vi "Close.vi"(8 "error in (no error)":errorcluster, 11 "Accelerometer Ref In":T1) -> (0 "error out":errorcluster)   [LabVIEW 2021, in "Accelerometer.lvlib"]
doc: "Closes the reference to accelerometer channels."
uses:
  <vilib>/myRIO/Instrument Drivers/Onboard Devices/Accelerometer/Accelerometer.lvlib
  <vilib>/myRIO/Instrument Drivers/Onboard Devices/Accelerometer/typedefs/Accelerometer Reference.ctl
  <vilib>/myRIO/Common/Instrument Driver Framework/Utilities/typedefs/myRIO Generic Hardware Reference.ctl
  <vilib>/myRIO/Common/Instrument Driver Framework/Utilities/typedefs/Hardware Version Enum.ctl
  <vilib>/myRIO/Common/Instrument Driver Framework/Utilities/typedefs/myRIO v1.0 Reference.ctl
  <vilib>/myRIO/Common/Instrument Driver Framework/Utilities/typedefs/Generic FPGA Reference.ctl
  <vilib>/myRIO/Common/Instrument Driver Framework/myRIO v1.0/Accelerometer/typedefs/Accelerometer Channels List.ctl
  <vilib>/myRIO/Common/Instrument Driver Framework/myRIO v1.0/Accelerometer/typedefs/Accelerometer Channels Enum.ctl
  <vilib>/myRIO/Common/Instrument Driver Framework/myRIO v1.0/Accelerometer/vis/myRIO v1.0 Unreserve Accelerometer.vi
  <vilib>/myRIO/Common/Instrument Driver Framework/roboRIO v1.0/Accelerometer/vis/roboRIO v1.0 Unreserve Accelerometer.vi
  <vilib>/myRIO/Common/Instrument Driver Framework/myRIO v1.0/Resource Manager/vis/myRIO v1.0 Unreserve Channel List.vi
  <vilib>/myRIO/Common/Instrument Driver Framework/myRIO v1.0/Accelerometer/vis/myRIO v1.0 Build MUX Configuration Accelerometer.vi
  <vilib>/myRIO/Common/Instrument Driver Framework/roboRIO v1.0/Resource Manager/vis/roboRIO v1.0 Unreserve Channel List.vi
  <vilib>/myRIO/Common/Instrument Driver Framework/roboRIO v1.0/Accelerometer/vis/roboRIO v1.0 Build MUX Configuration Accelerometer.vi
  <vilib>/myRIO/Common/Instrument Driver Framework/myRIO v1.0/Resource Manager/vis/myRIO v1.0 Unreserve Channel.vi
  <vilib>/myRIO/Common/Instrument Driver Framework/roboRIO v1.0/Resource Manager/vis/roboRIO v1.0 Unreserve Channel.vi
  <vilib>/myRIO/Common/Instrument Driver Framework/myRIO v1.0/Resource Manager/vis/myRIO v1.0 Build Mutex Name.vi
  <vilib>/myRIO/Common/Instrument Driver Framework/roboRIO v1.0/Resource Manager/vis/roboRIO v1.0 Build Mutex Name.vi
  <vilib>/myRIO/Common/Instrument Driver Framework/Utilities/vis/Configuration Manager.vi
  <vilib>/myRIO/Common/Instrument Driver Framework/Utilities/vis/IO Manager.vi
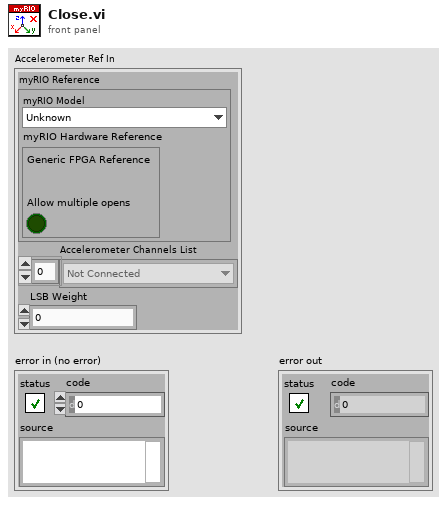
[diagram p1: front panel]
types:
  T1 = typedef "Accelerometer.lvlib/Accelerometer Reference.ctl" = cluster{"myRIO Reference":T2, "Accelerometer Channels List":T6, "LSB Weight":dbl}
  T2 = typedef "myRIO Generic Hardware Reference.ctl" = cluster{"myRIO Model":T3, "myRIO Hardware Reference":T4}
  T3 = typedef "Hardware Version Enum.ctl" = enum16{"Unknown", "myRIO-1900", "myRIO-1950", "roboRIO", "NI ELVIS RIO CM", "ELVIS III"}
  T4 = typedef "myRIO v1.0 Reference.ctl" = cluster{"Generic FPGA Reference":T5, "Allow multiple opens":bool}
  T5 = typedef "Generic FPGA Reference.ctl" = refnum<k20>
  T6 = typedef "Accelerometer Channels List.ctl" = T7[]
  T7 = typedef "Accelerometer Channels Enum.ctl" = enum16{"Not Connected", "X-Axis", "Y-Axis", "Z-Axis"}
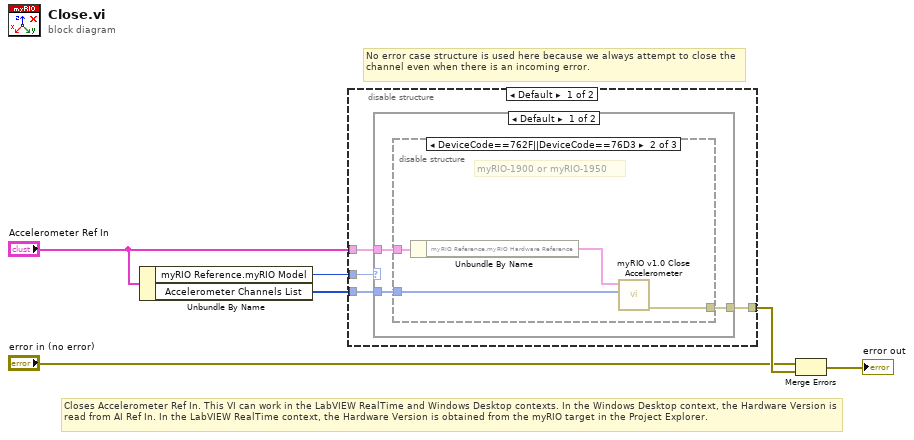
[diagram p0: block diagram]
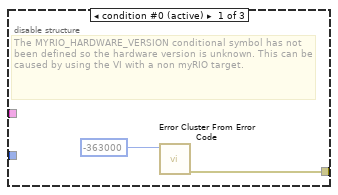
[diagram p2: hidden frame]
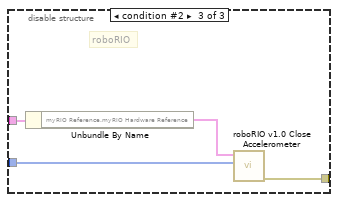
[diagram p3: hidden frame]
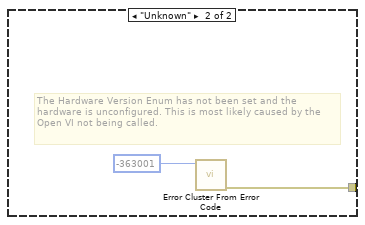
[diagram p4: hidden frame]
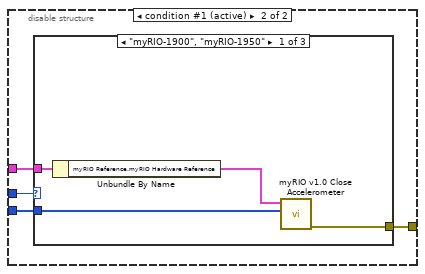
[diagram p5: hidden frame]
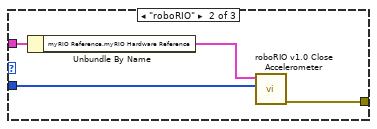
[diagram p6: hidden frame]
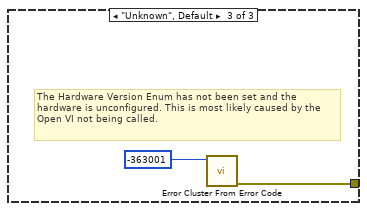
[diagram p7: hidden frame]
diagram:
  # "No error case structure is used here because we always attempt to close the channel even when there is an incoming error."
  # "Closes Accelerometer Ref In. This VI can work in the LabVIEW RealTime and Windows Desktop contexts. In the Windows Desktop context, the Hardware Version is read from AI Ref In. In the LabVIEW RealTime context, the Hardware Version is obtained from the myRIO target in the Project Explorer."
  n1 = Unbundle By Name("Accelerometer Ref In") -> ("myRIO Reference.myRIO Model"=w2:T3, "Accelerometer Channels List"=w1:T6)
  n2 = disable-structure shown="Default" {
    disable-tunnel: "Accelerometer Ref In" -> [w10 w28]
    disable-tunnel: [w9 w29] -> w6
    disable-tunnel: w2 -> [w8 w27]
    disable-tunnel: w1 -> [w7 w26]
    frame condition #0 {
      n3 = case shown="Default" w8 {
        tunnel: w10 -> [w13 _]
        tunnel: [w12 w24] -> w9
        tunnel: w7 -> [w11 _]
        frame Default {
          n4 = disable-structure shown="DeviceCode==762F||DeviceCode==76D3" {
            disable-tunnel: w13 -> [_ w19 w23]
            disable-tunnel: [w14 w18 w22] -> w12
            disable-tunnel: w11 -> [_ w16 w20]
            frame condition #0 (active) {
              # "The MYRIO_HARDWARE_VERSION conditional symbol has not been defined so the hardware version is unknown. This can be caused by using the VI with a non myRIO target."
              n5 = call <vilib>:"Error Cluster From Error Code.vi"("error code (0)"=-363000) -> ("error out"=w14:errorcluster)  [unwired: 8 in]
            }
            frame condition #1 {
              # "myRIO-1900 or myRIO-1950"
              n6 = Unbundle By Name(w19) -> ("myRIO Reference.myRIO Hardware Reference"=w17:T4)
              n7 = call <vilib>:"myRIO v1.0 Close Accelerometer.vi"("Accelerometer Channel List"=w16, "myRIO Ref In"=w17) -> ("error out"=w18:errorcluster)  [unwired: 9 in]
            }
            frame condition #2 {
              # "roboRIO"
              n8 = Unbundle By Name(w23) -> ("myRIO Reference.myRIO Hardware Reference"=w21:T4)
              n9 = call <vilib>:"roboRIO v1.0 Close Accelerometer.vi"("Accelerometer Channel List"=w20, "myRIO Ref In"=w21) -> ("error out"=w22:errorcluster)  [unwired: 9 in]
            }
          }
        }
        frame "Unknown" {
          # "The Hardware Version Enum has not been set and the hardware is unconfigured. This is most likely caused by the Open VI not being called."
          n10 = call <vilib>:"Error Cluster From Error Code.vi"("error code (0)"=-363001) -> ("error out"=w24:errorcluster)  [unwired: 8 in]
        }
      }
    }
    frame condition #1 (active) {
      n11 = case shown="\"myRIO-1900\", \"myRIO-1950\"" w27 {
        tunnel: w28 -> [w33 w37 _]
        tunnel: [w32 w36 w38] -> w29
        tunnel: w26 -> [w30 w34 _]
        frame "myRIO-1900", "myRIO-1950" {
          n12 = Unbundle By Name(w33) -> ("myRIO Reference.myRIO Hardware Reference"=w31:T4)
          n13 = call <vilib>:"myRIO v1.0 Close Accelerometer.vi"("Accelerometer Channel List"=w30, "myRIO Ref In"=w31) -> ("error out"=w32:errorcluster)  [unwired: 9 in]
        }
        frame "roboRIO" {
          n14 = Unbundle By Name(w37) -> ("myRIO Reference.myRIO Hardware Reference"=w35:T4)
          n15 = call <vilib>:"roboRIO v1.0 Close Accelerometer.vi"("Accelerometer Channel List"=w34, "myRIO Ref In"=w35) -> ("error out"=w36:errorcluster)  [unwired: 9 in]
        }
        frame "Unknown", Default {
          # "The Hardware Version Enum has not been set and the hardware is unconfigured. This is most likely caused by the Open VI not being called."
          n16 = call <vilib>:"Error Cluster From Error Code.vi"("error code (0)"=-363001) -> ("error out"=w38:errorcluster)  [unwired: 8 in]
        }
      }
    }
  }
  n17 = Merge Errors("error in (no error)", w6) -> (→"error out":errorcluster)
